vi "AlliGator Sliced Mean, SDV & CV Plots Event.vi"(8 "Error In":errorcluster, 10 "Mouse Coordinates":T1, 11 "Multiplot XY Graph":T2) -> (0 "Error Out":errorcluster, 1 "Message":string)   [LabVIEW 2021, in "AlliGator Lifetime & Other Parameters.lvlib"]
uses:
  AlliGator Lifetime & Other Parameters.lvlib
  Graphs/XY Graph/XY Graph Refnum.ctl
  <vilib>/Utility/miscctls.llb/LVPoint32TypeDef.ctl
  Graphs/Get Plot at Mouse Click (XY Graph)/Get Plot at Mouse Click [AAC].vi
  Graphs/Graphs.lvlib
  Variant/Variant.lvlib
  Graphs/XY Graph/XY Graph Add-Ons.lvlib
panel:
  # "see the License on the block diagram (Ctrl+E or Window:Show Block Diagram)"
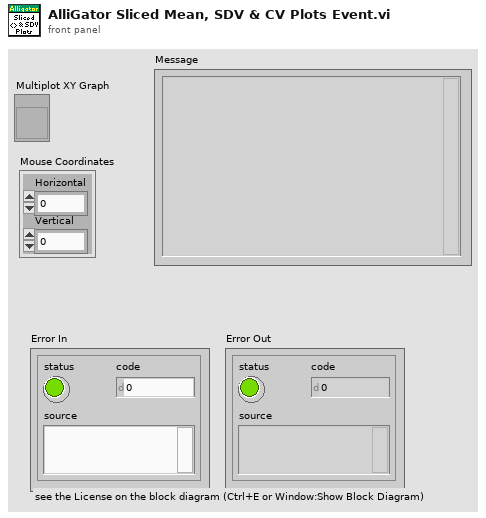
[diagram p1: front panel]
types:
  T1 = typedef "LVPoint32TypeDef.ctl" = cluster{"Horizontal":i32, "Vertical":i32}
  T2 = typedef "XY Graph Add-Ons.lvlib/XY Graph Refnum.ctl" = refnum<vi>
  T3 = typedef "XY Graph Add-Ons.lvlib/XY Graph Sliced Mean & SDV Step Definition.ctl" = cluster{"Axis Start":dbl, "Axis Stop":dbl, "# Steps":i32, "Step Size":dbl, "Step Definition":T4, "Upper Percentile":dbl, "Lower Percentile":dbl, "Min # Data Points/Slice":i32, "Output Abscissa Statistics Plots":bool, "Bin Location":T5, "# Elements":i32, "Bootstrap CV's SDV":bool, "# Replicas":i32}
  T4 = typedef "AlliGator Lifetime & Other Parameters.lvlib/AlliGator Intensity Slice Definition.ctl" = enum32{"# Steps", "Step Size", "# Elements"}
  T5 = typedef "XY Graph Add-Ons.lvlib/XY Graph Sliced CV Abscissa Location.ctl" = enum16{"Left", "Center", "Mean", "Right"}
  T6 = typedef "AlliGator Decay Fit Parameter Map.lvlib/AlliGator Sliced Analysis Plots.ctl" = cluster{"[<tau>(I)]":T7, "[SDV(tau)(I)]":T7, "[CV(tau)(I)]":T7, "[CV(tau)(I) SDV]":T7, "[N(I)]":T7, "[<I>(I)]":T7, "[SDV(I)(I)]":T7}
  T7 = typedef "XY Graph Add-Ons.lvlib/XY Graph Plot Data.ctl" = cluster{"X Array":dbl[], "Y Array":dbl[]}
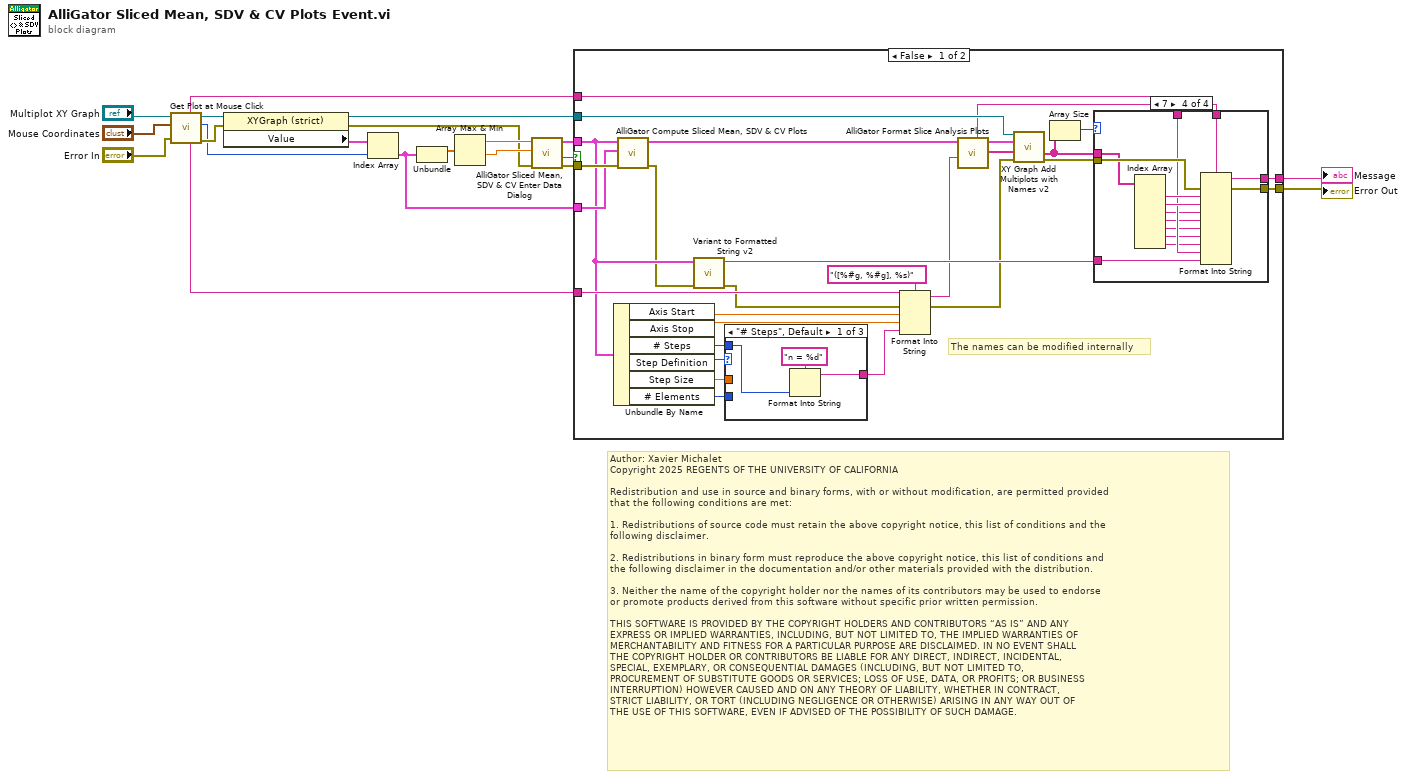
[diagram p0: block diagram]
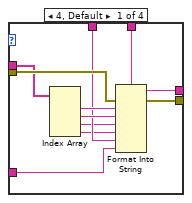
[diagram p2: hidden frame]
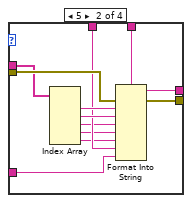
[diagram p3: hidden frame]
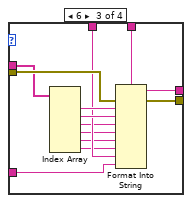
[diagram p4: hidden frame]
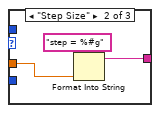
[diagram p5: hidden frame]
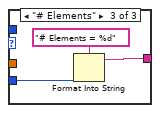
[diagram p6: hidden frame]
diagram:
  # "Author: Xavier Michalet\nCopyright 2025 REGENTS OF THE UNIVERSITY OF CALIFORNIA\n\nRedistribution and use in source and binary forms, with or without modification, are permitted provided\nthat the following conditions are met:\n\n1. Redistributions of source code must retain the above copyright notice, this list of conditions and the\nfollowing disclaimer.\n\n2. Redistributions in binary form must reproduce the above copyright notice, this list of conditions and\nthe following disclaimer in the documentation and/or other materials provided with the distribution.\n\n3. Neither the name of the copyright holder nor the names of its contributors may be used to endorse \nor promote products derived from this software without specific prior written permission.\n\nTHIS SOFTWARE IS PROVIDED BY THE COPYRIGHT HOLDERS AND CONTRIBUTORS “AS IS” AND ANY \nEXPRESS OR IMPLIED WARRANTIES, INCLUDING, BUT NOT LIMITED TO, THE IMPLIED WARRANTIES OF\nMERCHANTABILITY AND FITNESS FOR A PARTICULAR PURPOSE ARE DISCLAIMED. IN NO EVENT SHALL\nTHE COPYRIGHT HOLDER OR CONTRIBUTORS BE LIABLE FOR ANY DIRECT, INDIRECT, INCIDENTAL, \nSPECIAL, EXEMPLARY, OR CONSEQUENTIAL DAMAGES (INCLUDING, BUT NOT LIMITED TO, \nPROCUREMENT OF SUBSTITUTE GOODS OR SERVICES; LOSS OF USE, DATA, OR PROFITS; OR BUSINESS\nINTERRUPTION) HOWEVER CAUSED AND ON ANY THEORY OF LIABILITY, WHETHER IN CONTRACT, \nSTRICT LIABILITY, OR TORT (INCLUDING NEGLIGENCE OR OTHERWISE) ARISING IN ANY WAY OUT OF\nTHE USE OF THIS SOFTWARE, EVEN IF ADVISED OF THE POSSIBILITY OF SUCH DAMAGE."
  n1 = call-poly "Get Plot at Mouse Click.vi"("error in (no error)"="Error In", "Mouse Click Coordinates"="Mouse Coordinates", "XY Graph in"="Multiplot XY Graph") -> ("error out"=w18:errorcluster, "Plot at Coordinates"=w16:i32, "XY Graph out"=w19:T2, "Plot Name"=w4:string, "Graph Name"=w14:string)  [unwired: 2 in, 2 out]
  n2 = property class="XYGraph (strict)"(reference=w19, error in=w18) -> (reference out=w15:T2, error out=w8:errorcluster, "Value"=w17:cluster{"X Array":dbl[], "Y Array":dbl[]}[])
  n3 = Index Array(array=w17, index=w16) -> (element=w6:cluster{"X Array":dbl[], "Y Array":dbl[]})
  n4 = Unbundle(w6) -> ("X Array"=w11:dbl[])  [unwired: 1 out]
  n5 = Array Max & Min(array=w11) -> (max value=w10:dbl, min value=w9:dbl)  [unwired: 2 out]
  n6 = call "AlliGator Sliced Mean, SDV & CV Enter Data Dialog.vi"("Error In"=w8, "X min"=w9, "X max"=w10) -> ("Error Out"=w7:errorcluster, "Cancelled?"=w1:bool, "Slices Definition out"=w5:T3)  [unwired: 6 in]
  n7 = case shown="False" w1 {
    tunnel: w15 -> [w48 _]
    tunnel: w14 -> [w37 _]
    tunnel: [w46 _] -> w13
    tunnel: [w45 w108] -> w12
    tunnel: w7 -> [w44 w108]
    tunnel: w6 -> [w43 _]
    tunnel: w5 -> [w33 _]
    tunnel: w4 -> [w42 _]
    frame False {
      # "The names can be modified internally"
      n8 = Unbundle By Name(w33) -> ("Axis Start"=w36:dbl, "Axis Stop"=w35:dbl, "# Steps"=w39:i32, "Step Definition"=w40:T4, "Step Size"=w38:dbl, "# Elements"=w21:i32)
      n9 = call "AlliGator Compute Sliced Mean, SDV & CV Plots.vi"("error in (no error)"=w44, "tau(I) Plot"=w43, "Slices Definition"=w33) -> ("error out"=w30:errorcluster, "Result Plots Cluster"=w28:T6)  [unwired: 5 in, 2 out]
      n10 = call "Variant to Formatted String v2.vi"("error in (no error)"=w30, "Anything"=w33) -> ("error out"=w32:errorcluster, "String"=w31:string)  [unwired: 8 in]
      n11 = case shown="\"# Steps\", Default" w40 {
        tunnel: w39 -> [w101 _ _]
        tunnel: [w99 w103 w106] -> w34
        tunnel: w38 -> [_ w102 _]
        tunnel: w21 -> [_ _ w105]
        frame "# Steps", Default {
          n12 = Format Into String(format string="n = %d", w101) -> (resulting string=w99:string)  [unwired: 2 in, 1 out]
        }
        frame "Step Size" {
          n13 = Format Into String(format string="step = %#g", w102) -> (resulting string=w103:string)  [unwired: 2 in, 1 out]
        }
        frame "# Elements" {
          n14 = Format Into String(format string="# Elements = %d", w105) -> (resulting string=w106:string)  [unwired: 2 in, 1 out]
        }
      }
      n15 = Format Into String(format string="([%#g, %#g], %s)", initial string=w42, error in=w32, w36, w35, w34) -> (resulting string=w29:string, error out=w22:errorcluster)
      n16 = call "AlliGator Format Slice Analysis Plots.vi"("Plot Name Suffix"=w29, "Result Plots Cluster"=w28) -> ("Array of Plot Names"=w23:string[], "Array of Plots"=w24:cluster{"X Array":dbl[], "Y Array":dbl[]}[], "format string"=w27:string)  [unwired: 7 in]
      n17 = call "XY Graph Add Multiplots with Names v2.vi"("XYGraph in"=w48, "Array of Plots"=w24, "Array of Plot Names (\"Plot\")"=w23, "error in (no error)"=w22) -> ("Added Plot Names"=w26:string[], "error out"=w47:errorcluster)  [unwired: 7 in, 3 out]
      n18 = Array Size(array=w26) -> (size(s)=w25:i32)
      n19 = case shown="7" w25 {
        tunnel: w47 -> [w59 w71 w84 w98]
        tunnel: [w58 w70 w83 w97] -> w46
        tunnel: [w57 w69 w82 w96] -> w45
        tunnel: w26 -> [w56 w68 w81 w95]
        tunnel: w37 -> [w53 w65 w78 w92]
        tunnel: w31 -> [w51 w63 w76 w90]
        tunnel: w27 -> [w50 w62 w75 w89]
        frame 4, Default {
          n20 = Index Array(array=w56) -> (element #1=w55:string, element #2=w54:string, element #3=w52:string, element #4=w49:string)  [unwired: 4 in]
          n21 = Format Into String(format string=w50, error in=w59, w55, w54, w52, w49, w53, w51) -> (resulting string=w58:string, error out=w57:errorcluster)  [unwired: 1 in]
        }
        frame 5 {
          n22 = Index Array(array=w68) -> (element #1=w67:string, element #2=w66:string, element #3=w64:string, element #4=w61:string, element #5=w60:string)  [unwired: 5 in]
          n23 = Format Into String(format string=w62, error in=w71, w67, w66, w64, w61, w60, w65, w63) -> (resulting string=w70:string, error out=w69:errorcluster)  [unwired: 1 in]
        }
        frame 6 {
          n24 = Index Array(array=w81) -> (element #1=w80:string, element #2=w79:string, element #3=w77:string, element #4=w74:string, element #5=w73:string, element #6=w72:string)  [unwired: 6 in]
          n25 = Format Into String(format string=w75, error in=w84, w80, w79, w77, w74, w73, w72, w78, w76) -> (resulting string=w83:string, error out=w82:errorcluster)  [unwired: 1 in]
        }
        frame 7 {
          n26 = Index Array(array=w95) -> (element #1=w94:string, element #2=w93:string, element #3=w91:string, element #4=w88:string, element #5=w87:string, element #6=w86:string, element #7=w85:string)  [unwired: 7 in]
          n27 = Format Into String(format string=w89, error in=w98, w94, w93, w91, w88, w87, w86, w85, w92, w90) -> (resulting string=w97:string, error out=w96:errorcluster)  [unwired: 1 in]
        }
      }
    }
    frame True {
      # "Cancelled"
    }
  }
  "Error Out" <- w12
  "Message" <- w13
